vi "Srednia PBP.vi"(9 "Srednia N-1":dbl, 10 "N":i32, 11 "Punkty":dbl) -> (3 "Srednia":dbl)   [LabVIEW 2019]
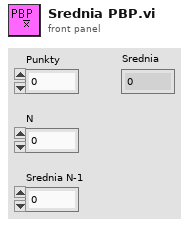
[diagram p1: front panel]
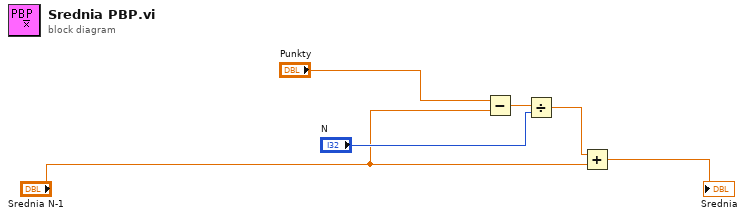
[diagram p0: block diagram]
diagram:
  n1 = Subtract(x="Punkty", y="Srednia N-1") -> (x-y=w2:dbl)
  n2 = Divide(x=w2, y="N") -> (x/y=w4:dbl)
  n3 = Add(x=w4, y="Srednia N-1") -> (x+y=→"Srednia":dbl)
